vi "qp_manage working set.vi"(0 "working set indices in":i32[](array[numeric]), 1 "A working set":T2, 2 "b working set":dbl[](array[numeric]), 3 "not working set indices in":i32[](array[numeric]), 4 "A not working set":T2, 5 "b not working set":dbl[](array[numeric]), 9 "index":i32, 11 "direction":T1(radio)) -> (14 "working set indices out":i32[](array[numeric]), 15 "A working set":T2, 16 "b working set":dbl[](array[numeric]), 17 "not working set indices out":i32[](array[numeric]), 18 "A not working set":T2, 19 "b not working set":dbl[](array[numeric]))   [LabVIEW 2017, in "NI_Gmath.lvlib"]
uses:
  <vilib>/gmath/NI_Gmath.lvlib
  <vilib>/Analysis/Matrix/Datatypes/RealMatrix.ctl
  <vilib>/Analysis/Matrix/NI_Matrix.lvlib
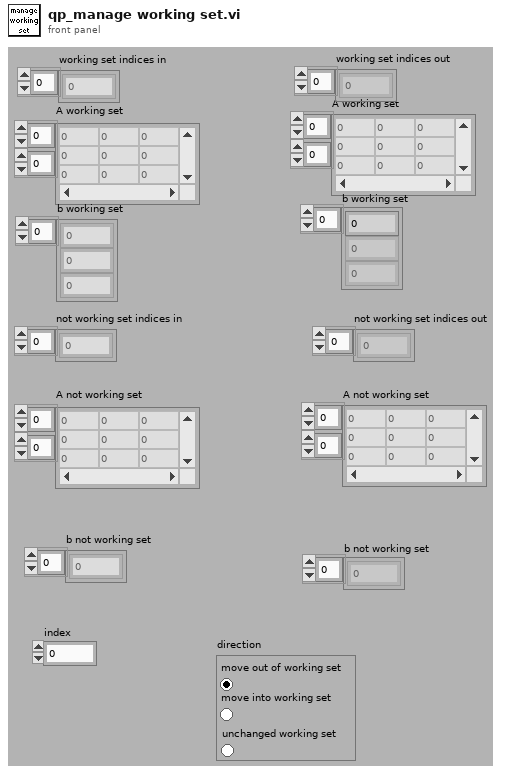
[diagram p1: front panel]
types:
  T1 = enum32{"move out of working set", "move into working set", "unchanged working set"}
  T2 = typedef "NI_Matrix.lvlib/RealMatrix.ctl" = dbl[][]
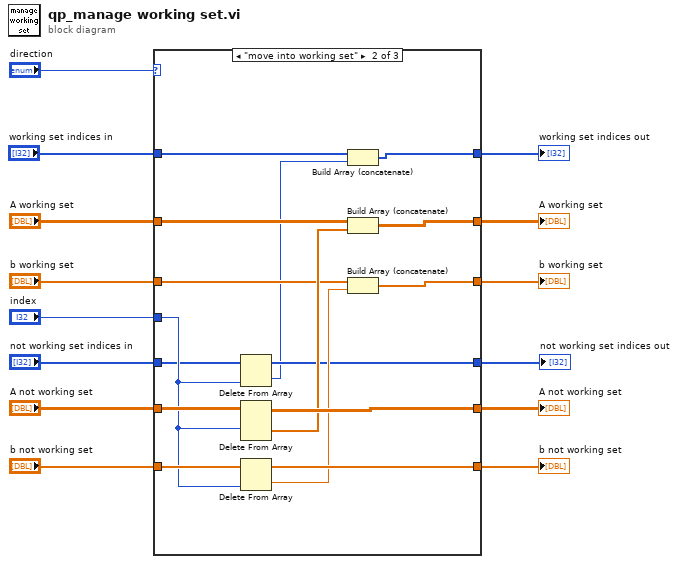
[diagram p0: block diagram]
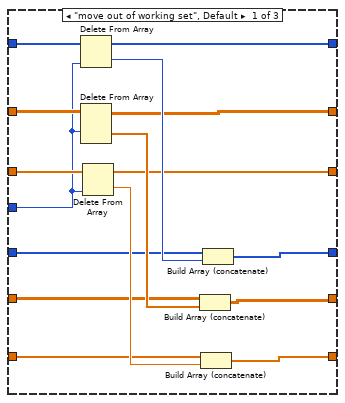
[diagram p2: hidden frame]
diagram:
  n1 = case shown="\"move into working set\"" "direction" {
    tunnel: "A working set" -> [w26 w42 w52]
    tunnel: "b working set" -> [w24 w39 w51]
    tunnel: "A not working set" -> [w22 w46 w50]
    tunnel: "b not working set" -> [w21 w45 w49]
    tunnel: [w25 w40 w52] -> w12
    tunnel: [w23 w37 w51] -> w11
    tunnel: [w28 w44 w50] -> w10
    tunnel: [w20 w43 w49] -> w9
    tunnel: "index" -> [w15 w34 _]
    tunnel: "working set indices in" -> [w17 w36 w48]
    tunnel: "not working set indices in" -> [w19 w33 w47]
    tunnel: [w18 w32 w47] -> w2
    tunnel: [w16 w35 w48] -> w1
    frame "move out of working set", Default {
      n2 = Delete From Array(array=w17, index=w15) -> (deleted portion=w30:i32, array with subset deleted=w16:i32[])  [unwired: 1 in]
      n3 = Delete From Array(array=w26, index (row)=w15) -> (deleted portion=w27:dbl[], array with subset deleted=w25:T2)  [unwired: 2 in]
      n4 = Delete From Array(array=w24, index=w15) -> (deleted portion=w29:dbl, array with subset deleted=w23:dbl[])  [unwired: 1 in]
      n5 = Build Array (concatenate)(w22, w27) -> (w28:T2)
      n6 = Build Array (concatenate)(w21, w29) -> (w20:dbl[])
      n7 = Build Array (concatenate)(w19, w30) -> (w18:i32[])
    }
    frame "move into working set" {
      n8 = Delete From Array(array=w33, index=w34) -> (deleted portion=w31:i32, array with subset deleted=w32:i32[])  [unwired: 1 in]
      n9 = Delete From Array(array=w46, index (row)=w34) -> (deleted portion=w41:dbl[], array with subset deleted=w44:T2)  [unwired: 2 in]
      n10 = Delete From Array(array=w45, index=w34) -> (deleted portion=w38:dbl, array with subset deleted=w43:dbl[])  [unwired: 1 in]
      n11 = Build Array (concatenate)(w36, w31) -> (w35:i32[])
      n12 = Build Array (concatenate)(w42, w41) -> (w40:T2)
      n13 = Build Array (concatenate)(w39, w38) -> (w37:dbl[])
    }
    frame "unchanged working set" {
    }
  }
  "A working set" <- w12
  "b working set" <- w11
  "A not working set" <- w10
  "b not working set" <- w9
  "working set indices out" <- w1
  "not working set indices out" <- w2
